vi "Set Value.vi"(8 "error in (no error)":errorcluster, 9 "value":string, 10 "name":string, 11 "Keyed Value Tree in":refnum<class "Keyed Value Tree.lvclass">) -> (0 "error out":errorcluster, 2 "replaced":bool, 3 "Keyed Value Tree out":refnum<class "Keyed Value Tree.lvclass">)   [LabVIEW 2027, in "Keyed Value Tree.lvclass"]
uses:
  Keyed Value Tree.lvclass
  Keyed Value Tree.lvclass/Keyed Value Tree.ctl
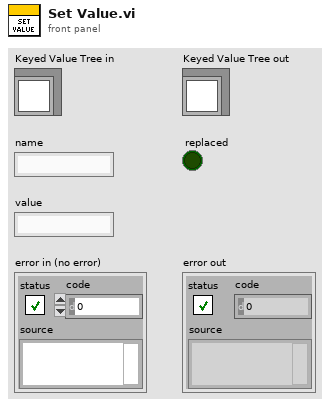
[diagram p1: front panel]
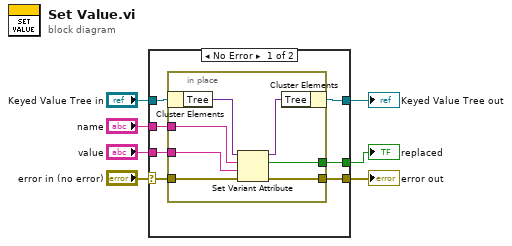
[diagram p0: block diagram]
diagram:
  n1 = case shown="No Error" "error in (no error)" {
    selector: "error in (no error)" -> [w9 w23]
    tunnel: [w8 w23] -> w6
    tunnel: [w13 w22] -> w4
    tunnel: "Keyed Value Tree in" -> [w14 w22]
    tunnel: "value" -> [w12 _]
    tunnel: "name" -> [w11 _]
    tunnel: [w10 _] -> w1
    frame No Error {
      n2 = in-place {
        in-place-border: w12 -> [w19]
        in-place-border: w11 -> [w18]
        in-place-border: [w17] -> w10
        in-place-border: w9 -> [w16]
        in-place-border: [w15] -> w8
        n3 = in-place-cluster #1(w14) -> ("Tree"=w21:variant)
        n4 = Set Variant Attribute(Variant=w21, name=w18, value=w19, error in=w16) -> (Variant out=w20:variant, replaced=w17:bool, error out=w15:errorcluster)
        n5 = in-place-cluster #1("Tree"=w20) -> (w13:refnum<class "Keyed Value Tree.lvclass">)
      }
    }
    frame Error {
    }
  }
  "error out" <- w6
  "Keyed Value Tree out" <- w4
  "replaced" <- w1
